vi "CPP-ZeroMaintenance.vi"(1 "SecondsToAverage":dbl=10.0, 2 "SecondsToMonitor":dbl=30.0, 3 "Tunnel#:Pressures:":string="Tunnel3:Pressures:") -> (0 "Time Elapsed since zero (min)":dbl format="%#.2f")   [LabVIEW 2014]
doc: "This VI monitors an array of Tunnel Pressures Depending on the input \"Tunnel#:Pressures:\" (e.g. appropriate inputs are \"Tunnel1:Pressures:\" and \"Tunnel3:Pressures:\"). \"SecondsToMonitor\" is the interval used to determine whether the tunnel has been off long enough, and \"SecondsToAverage\" is the averaging interval for recording zeros."
uses:
  Sub VIs/ADAM Controls/Ch_description_ADAM.ctl
  Sub VIs/ADAM Controls/Module_type_ADAM.ctl
  Sub VIs/ADAM Controls/Function_ADAM.ctl
  Sub VIs/ADAM Controls/Channel_State.ctl
  Sub VIs/ADAM Controls/Calib_type_ADAM.ctl
  Sub VIs/ADAM Controls/Address.ctl
panel:
  out "Listening Value":dbl=0.2694398123338766
  out "Old Zero time":dbl=3521053410.165856 format="%#.0f"
  out "current time":timestamp=timestamp(3521053420.076362 s since 1904-01-01)
  out "Current Time (sec)":dbl=3521053420.076362 format="%#.0f"
  out "New Zero Time":dbl=3521053420.076362 format="%#.0f"
  in  "Threshold: Listening Channel":dbl=1.0 format="%#_13g"
  in  "Monitored Tunnel Pressures":T1(tab)=enum."Tunnel3:Pressures:"
  in  "ADAM Ch Names: Tunnel 1":string[](array[string])=["Tunnel1:StaticP:0", "Tunnel1:StaticP:1", "Tunnel1:StaticP:2", "Tunnel1:StaticP:3", "Tunnel1:StaticP:4", "Tunnel1:StaticP:5", "Tunnel1:StaticP:6", "Tunnel1:StaticP:7"]
  in  "ADAM Ch Names: Tunnel 3":string[](array[string])=["Tunnel3:StaticP:0", "Tunnel3:StaticP:1", "Tunnel3:StaticP:2", "Tunnel3:StaticP:3", "Tunnel3:StaticP:4", "Tunnel3:StaticP:5", "Tunnel3:StaticP:6", "Tunnel3:StaticP:7", "Tunnel3:StaticP:8", "Tunnel3:StaticP:+Fan"]
  out "Ch Description Array":T2[](array[typedef])=[{"Ch Name"="Tunnel3:StaticP:0", "Type"="Run VI Named:", "Function"=enum."Analogue Input", "Ch State"=enum."On", "Calibration type"=enum."Bx + A", "A"=1.7148751842084184, "B"=32.003, "C"=0.0, "D"=0.0, "Comments"="LabJackT7.vi", "Address"={"Main"=502, "Ch."=5, "Sub"=0, "Port Name"="192.168.124.53"}, "String"="TX1", "Duty"=65535}, {"Ch Name"="Tunnel3:StaticP:1", "Type"="Run VI Named:", "Function"=enum."Analogue Input", "Ch State"=enum."On", "Calibration type"=enum."Bx + A", "A"=2.284955144207084, "B"=31.694, "C"=0.0, "D"=0.0, "Comments"="LabJackT7.vi", "Address"={"Main"=502, "Ch."=4, "Sub"=0, "Port Name"="192.168.124.53"}, "String"="TX1", "Duty"=65535}, {"Ch Name"="Tunnel3:StaticP:2", "Type"="Run VI Named:", "Function"=enum."Analogue Input", "Ch State"=enum."On", "Calibration type"=enum."Bx + A", "A"=0.8167514317763294, "B"=31.181, "C"=0.0, "D"=0.0, "Comments"="LabJackT7.vi", "Address"={"Main"=502, "Ch."=6, "Sub"=0, "Port Name"="192.168.124.53"}, "String"="TX3", "Duty"=65535}, {"Ch Name"="Tunnel3:StaticP:3", "Type"="Run VI Named:", "Function"=enum."Analogue Input", "Ch State"=enum."On", "Calibration type"=enum."Bx + A", "A"=0.17846746627890178, "B"=32.393, "C"=0.0, "D"=0.0, "Comments"="LabJackT7.vi", "Address"={"Main"=502, "Ch."=7, "Sub"=0, "Port Name"="192.168.124.53"}, "String"="TX5", "Duty"=65535}, {"Ch Name"="Tunnel3:StaticP:4", "Type"="Run VI Named:", "Function"=enum."Analogue Input", "Ch State"=enum."On", "Calibration type"=enum."Bx + A", "A"=-0.7455541200451542, "B"=31.833, "C"=0.0, "D"=0.0, "Comments"="LabJackT7.vi", "Address"={"Main"=502, "Ch."=8, "Sub"=0, "Port Name"="192.168.124.53"}, "String"="TX7", "Duty"=65535}, {"Ch Name"="Tunnel3:StaticP:5", "Type"="Run VI Named:", "Function"=enum."Analogue Input", "Ch State"=enum."On", "Calibration type"=enum."Bx + A", "A"=1.7337124103296127, "B"=31.692, "C"=0.0, "D"=0.0, "Comments"="LabJackT7.vi", "Address"={"Main"=502, "Ch."=9, "Sub"=0, "Port Name"="192.168.124.53"}, "String"="TX9", "Duty"=65535}, {"Ch Name"="Tunnel3:StaticP:6", "Type"="Run VI Named:", "Function"=enum."Analogue Input", "Ch State"=enum."On", "Calibration type"=enum."Bx + A", "A"=1.7416261176572003, "B"=31.922, "C"=0.0, "D"=0.0, "Comments"="LabJackT7.vi", "Address"={"Main"=502, "Ch."=10, "Sub"=0, "Port Name"="192.168.124.53"}, "String"="TX11", "Duty"=65535}, {"Ch Name"="Tunnel3:StaticP:7", "Type"="Run VI Named:", "Function"=enum."Analogue Input", "Ch State"=enum."On", "Calibration type"=enum."Bx + A", "A"=0.8789188613999486, "B"=31.887, "C"=0.0, "D"=0.0, "Comments"="LabJackT7.vi", "Address"={"Main"=502, "Ch."=11, "Sub"=0, "Port Name"="192.168.124.53"}, "String"="TX13", "Duty"=65535}, {"Ch Name"="Tunnel3:StaticP:8", "Type"="Run VI Named:", "Function"=enum."Analogue Input", "Ch State"=enum."On", "Calibration type"=enum."Bx + A", "A"=8.468861361036973, "B"=31.82, "C"=0.0, "D"=0.0, "Comments"="LabJackT7.vi", "Address"={"Main"=502, "Ch."=12, "Sub"=0, "Port Name"="192.168.124.53"}, "String"="TX15", "Duty"=65535}, {"Ch Name"="Tunnel3:StaticP:+Fan", "Type"="Run VI Named:", "Function"=enum."Analogue Input", "Ch State"=enum."On", "Calibration type"=enum."Bx + A", "A"=-1.1681921149610845, "B"=32.333, "C"=0.0, "D"=0.0, "Comments"="LabJackT7.vi", "Address"={"Main"=502, "Ch."=13, "Sub"=0, "Port Name"="192.168.124.53"}, "String"="TX1", "Duty"=65535}] {"Duty" format="%.0b"; "D" format="%#_5g"; "C" format="%#_5g"; "B" format="%#_5g"; "A" format="%#_5g"}
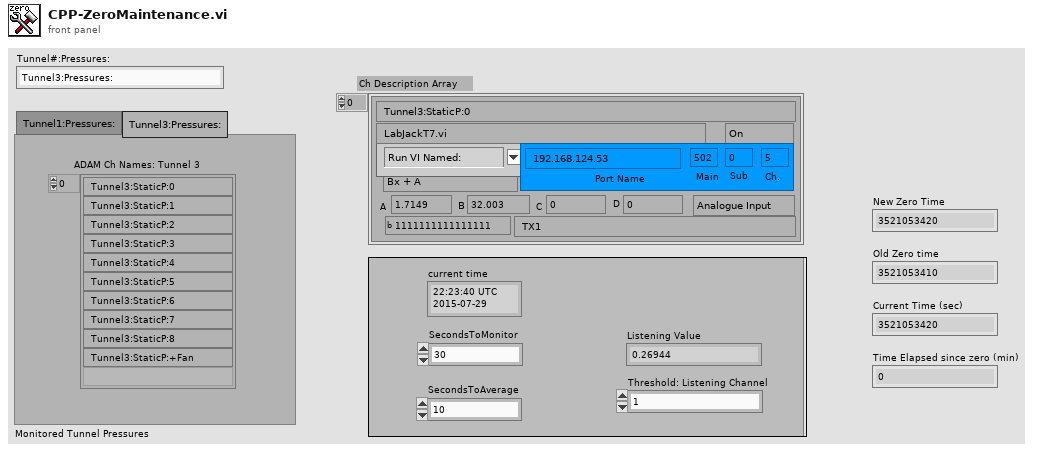
[diagram p1: front panel]
types:
  T1 = enum32{"Tunnel1:Pressures:", "Tunnel3:Pressures:"}
  T2 = typedef "Ch_description_ADAM.ctl" = cluster{"Ch Name":string, "Type":T3, "Function":T4, "Ch State":T5, "Calibration type":T6, "A":dbl, "B":dbl, "C":dbl, "D":dbl, "Comments":string, "Address":T7, "String":string, "Duty":u16}
  T3 = typedef "Module_type_ADAM.ctl" = string
  T4 = typedef "Function_ADAM.ctl" = enum16{"Analogue Input", "Digital Input", "Event counter", "Event rate", "Analogue Output", "Digital Output", "Relay Output"}
  T5 = typedef "Channel_State.ctl" = enum16{"On", "Off", "Always On", "Always Off"}
  T6 = typedef "Calib_type_ADAM.ctl" = enum16{"Raw", "Bx + A", "Cx^2 + Bx + A", "Dx^3 + Cx^2 + Bx + A", "In Band", "Hi-Tec Q", "Hi-Tec M_dot", "Text"}
  T7 = typedef "Address.ctl" = cluster{"Main":i32, "Ch.":i32, "Sub":i32, "Port Name":string}
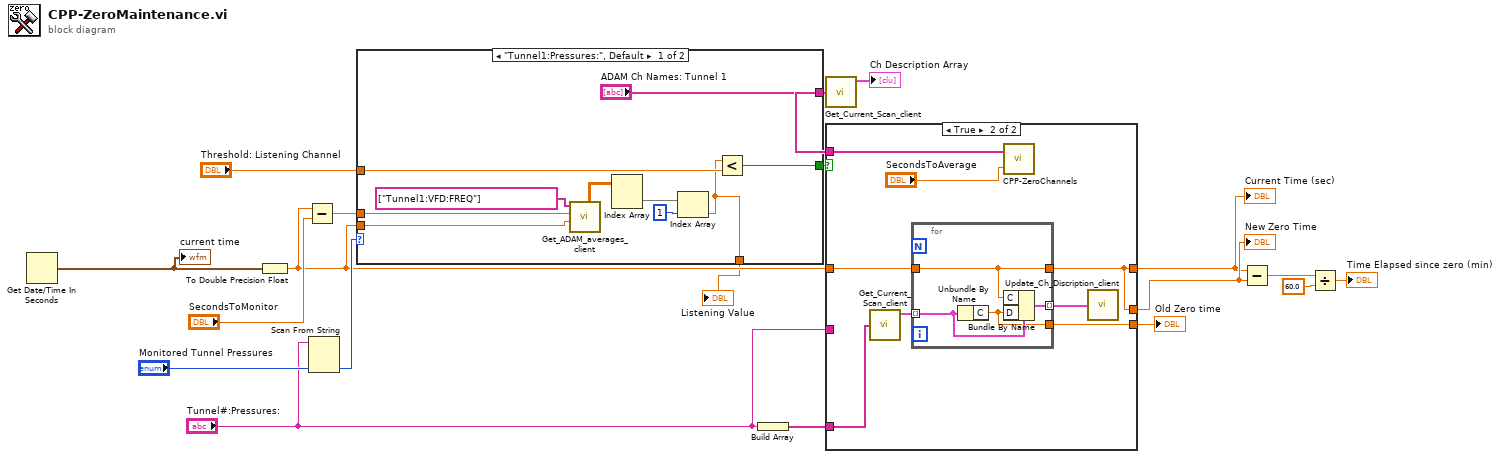
[diagram p0: block diagram]
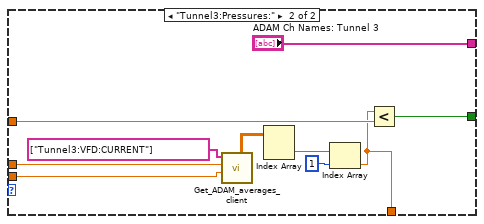
[diagram p2: hidden frame]
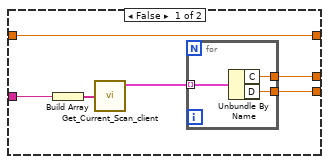
[diagram p3: hidden frame]
diagram:
  n1 = Get Date/Time In Seconds() -> (seconds since 1Jan1904=w19:timestamp)
  "current time" <- w19
  n2 = To Double Precision Float(number=w19) -> (double precision float=w4:dbl)
  n3 = Subtract(x=w4, y="SecondsToMonitor") -> (x-y=w5:dbl)
  n4 = Scan From String(input string="Tunnel#:Pressures:", default 1="Monitored Tunnel Pressures") -> (output 1=w14:T1)  [unwired: 3 in, 3 out]
  n5 = case shown="\"Tunnel1:Pressures:\", Default" w14 {
    tunnel: ["ADAM Ch Names: Tunnel 1" "ADAM Ch Names: Tunnel 3"] -> w17
    tunnel: w5 -> [w25 w38]
    tunnel: w4 -> [w24 w37]
    tunnel: [w21 w31] -> w3
    tunnel: "Threshold: Listening Channel" -> [w23 w32]
    tunnel: [w20 w30] -> w1
    frame "Tunnel1:Pressures:", Default {
      n6 = call "Get_ADAM_averages_client.vi"("End time"=w24, "Start time"=w25, "ADAM Ch Names"=string[] ["Tunnel1:VFD:FREQ"]) -> ("DBL values"=w26:dbl[][])  [unwired: 4 in, 4 out]
      n7 = Index Array(array=w26) -> (element=w28:dbl[])  [unwired: 2 in]
      n8 = Index Array(array=w28, index=1) -> (element=w20:dbl)
      n9 = Less?(x=w20, y=w23) -> (x < y?=w21:bool)
    }
    frame "Tunnel3:Pressures:" {
      n10 = call "Get_ADAM_averages_client.vi"("End time"=w37, "Start time"=w38, "ADAM Ch Names"=string[] ["Tunnel3:VFD:CURRENT"]) -> ("DBL values"=w36:dbl[][])  [unwired: 4 in, 4 out]
      n11 = Index Array(array=w36) -> (element=w34:dbl[])  [unwired: 2 in]
      n12 = Index Array(array=w34, index=1) -> (element=w30:dbl)
      n13 = Less?(x=w30, y=w32) -> (x < y?=w31:bool)
    }
  }
  "Listening Value" <- w1
  n14 = Build Array("Tunnel#:Pressures:") -> (w11:string[])
  n15 = call "Get_Current_Scan_client.vi"("ADAM Ch Names"=w17) -> ("Ch Description Array"=→"Ch Description Array":T2[])  [unwired: 3 out]
  n16 = case shown="True" w3 {
    tunnel: w17 -> [_ w56]
    tunnel: "Tunnel#:Pressures:" -> [w45 _]
    tunnel: [w42 w51] -> w13
    tunnel: w4 -> [w41 w53]
    tunnel: w11 -> [_ w52]
    tunnel: [w41 w51] -> w10
    tunnel: [w40 w50] -> w6
    frame False {
      n17 = Build Array(w45) -> (w44:string[])
      n18 = call "Get_Current_Scan_client.vi"("ADAM Ch Names"=w44) -> ("Ch Description Array"=w43:T2[])  [unwired: 3 out]
      n19 = for {
        tunnel: w43 -> [w48] mode=indexing
        tunnel: [w47] -> w42
        tunnel: [w46] -> w40
        n20 = Unbundle By Name(w48) -> ("C"=w47:dbl, "D"=w46:dbl)
      }
    }
    frame True {
      n21 = call "Get_Current_Scan_client.vi"("ADAM Ch Names"=w52) -> ("Ch Description Array"=w55:T2[])  [unwired: 3 out]
      n22 = for {
        tunnel: [w60] -> w54 mode=indexing
        tunnel: w55 -> [w59] mode=indexing
        tunnel: w53 -> [w58]
        tunnel: [w58] -> w51
        tunnel: [w57] -> w50
        n23 = Unbundle By Name(w59) -> ("C"=w57:dbl)
        n24 = Bundle By Name(cluster=w59, "C"=w58, "D"=w57) -> (w60:T2)
      }
      n25 = call "CPP-ZeroChannels.vi"("SecondsToAverage"="SecondsToAverage", "ADAM Ch Names"=w56) -> ()  [unwired: 1 out]
      n26 = call "Update_Ch_Discription_client.vi"("Channels to update In"=w54) -> ()  [unwired: 1 out]
    }
  }
  "New Zero Time" <- w13
  "Current Time (sec)" <- w10
  "Old Zero time" <- w6
  n27 = Subtract(x=w10, y=w13) -> (x-y=w9:dbl)
  n28 = Divide(x=w9, y=60.0) -> (x/y=→"Time Elapsed since zero (min)":dbl)
